vi "niRFUtil MEAS Max and Min (real array).vi"(2 "Real Array":T1 min=0 max=127 format="%.2f") -> (6 "Max":sgl format="%.2f", 7 "Min":sgl format="%.2f")   [LabVIEW 2015, in "niRFUtil.lvlib"]
doc: "(c) Copyright 2006, National Instruments, Inc. This VI may not be duplicated, sold, or distributed without written consent from National Instruments."
uses:
  niRFUtil.lvlib
  Includes/niRFUtil INC Real Array.ctl
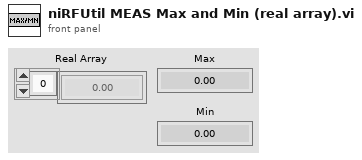
[diagram p1: front panel]
types:
  T1 = typedef "niRFUtil.lvlib/niRFUtil INC Real Array.ctl" = sgl[]
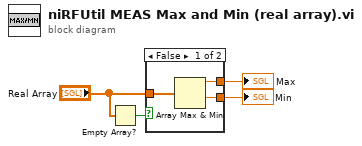
[diagram p0: block diagram]
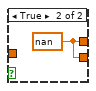
[diagram p2: hidden frame]
diagram:
  n1 = Empty Array?(array="Real Array") -> (empty?=w2:bool)
  n2 = case shown="False" w2 {
    tunnel: "Real Array" -> [w7 _]
    tunnel: [w6 w8] -> w4
    tunnel: [w5 w8] -> w3
    frame False {
      n3 = Array Max & Min(array=w7) -> (max value=w6:sgl, min value=w5:sgl)  [unwired: 2 out]
    }
    frame True {
      w8 = sgl nan
    }
  }
  "Max" <- w4
  "Min" <- w3
